vi "isRefValid.vi"(8 "error in (no error)":errorcluster, 11 "xwpfRun in":refnum<class "xwpfRun.lvclass">) -> (0 "error out":errorcluster, 3 "xwpfRun out":refnum<class "xwpfRun.lvclass">)   [LabVIEW 2017, in "Word_Specific.lvlib" / "xwpfRun.lvclass"]
uses:
  xwpfRun.lvclass
  xwpfRun.lvclass/xwpfRun.ctl
  <vilib>/Utility/error.llb/Error Cluster From Error Code.vi
  <vilib>/ErrorRing/Error Ring.xnode
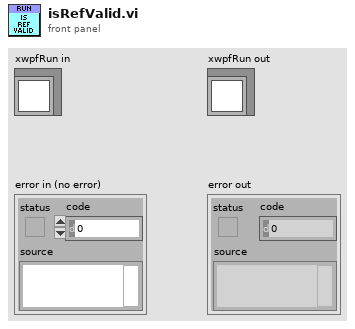
[diagram p1: front panel]
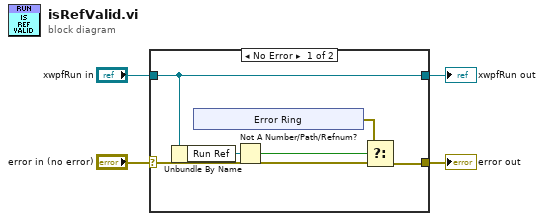
[diagram p0: block diagram]
diagram:
  n1 = case shown="No Error" "error in (no error)" {
    selector: "error in (no error)" -> [w6 w17]
    tunnel: [w5 w17] -> w3
    tunnel: [w9 w16] -> w1
    tunnel: "xwpfRun in" -> [w9 w16]
    frame No Error {
      n2 = Unbundle By Name(w9) -> ("Run Ref"=w10:refnum<k24>)
      n3 = xnode "Error Ring"() -> ("error out"=w7:errorcluster)
      n4 = Not A Number/Path/Refnum?(number/path/refnum=w10) -> (NaN/Path/Refnum?=w8:bool)
      n5 = Select(t=w7, s=w8, f=w6) -> (s? t:f=w5:errorcluster)
    }
    frame Error {
    }
  }
  "error out" <- w3
  "xwpfRun out" <- w1
